vi "Teleop.vi"(10 "Match Info":T2={"Autonomous Elapsed Seconds"=0.0, "TeleOp Elapsed Seconds"=72.02, "Disabled Elapsed Seconds"=100.939, "Visited Autonomous"=FALSE, "Visited TeleOp"=TRUE, "Visited Disabled"=TRUE, "Autonomous Settings"={"Autonomous Style"=enum."Independent", "VI Refnum"=refnum}}, 11 "Call Context":T3=enum."Stop") -> ()   [LabVIEW 2018]
doc: "This VI is called for each enabled TeleOp packet received from the DS. It is typically used to read from joysticks and other inputs and update I/O or setpoints for timed control loops. It should complete and return within 20 milliseconds or risk missing DS packets."
uses:
  <vilib>/Rock Robotics/WPI/DriverStation/WPI_DriverStationDerivedRobotMode.ctl
  <vilib>/Rock Robotics/WPI/DriverStation/WPI_DriverStationMatch Info.ctl
  Elevator/Implementation/Elevator Operations.ctl
  <vilib>/Rock Robotics/WPI/Utilities/WPI_GetSetVariantRefNum.vi
  Elevator/Implementation/Elevator Published Globals.vi
  <vilib>/Rock Robotics/Network Tables/NT Write Boolean.vi
  Framework/Robot Global Data.vi
  Configuration/Constants.vi
  <vilib>/Rock Robotics/Network Tables/NT Write Boolean Array.vi
  <vilib>/Rock Robotics/Network Tables/NT Write Numeric Array.vi
panel:
  in  "Anti-Gravity Elevator":dbl=0.06
  in  "Cluster":T1={"OutakeSpeed"=0.4, "OutakeSpeed Fast"=1.0, "Intake Sens"=1.2, "OutakeSens"=0.7} {"OutakeSpeed Fast" format="%#_13g"; "OutakeSpeed" format="%#_13g"}
  in  "ElevatorheightToSLowMode":dbl=25.0 format="%#_13g"
  in  "ElevatorInterpolate":cluster{"X":dbl, "Y":dbl}[](array[cluster])=[{"X"=0.0, "Y"=0.0}, {"X"=0.05, "Y"=0.0}, {"X"=0.8, "Y"=0.3}, {"X"=1.0, "Y"=1.0}]
  in  "ElevatorheightToSLowerMode":dbl=45.0 format="%#_13g"
  in  "Max dx/dt":dbl=100.0
  in  "Points":cluster{"X":dbl, "Y":dbl}[](array[cluster])=[{"X"=0.0, "Y"=0.0}, {"X"=0.02, "Y"=0.0}, {"X"=0.021, "Y"=0.15}, {"X"=1.0, "Y"=1.0}]
  in  "Drive":enum16{"Cheesy", "Tank"}(ring)
  # "Keep negative"
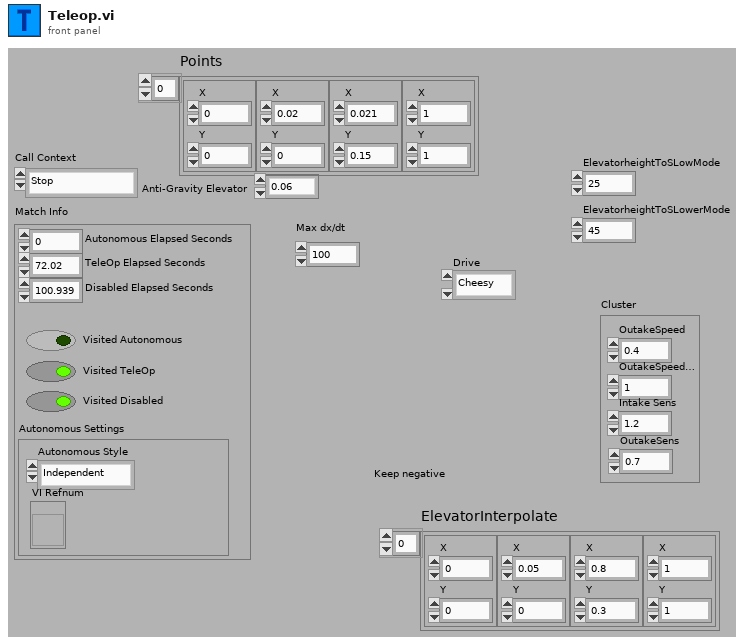
[diagram p1: front panel]
types:
  T1 = cluster{"OutakeSpeed":dbl, "OutakeSpeed Fast":dbl, "Intake Sens":dbl, "OutakeSens":dbl}
  T2 = typedef "WPI_DriverStationMatch Info.ctl" = cluster{"Autonomous Elapsed Seconds":dbl, "TeleOp Elapsed Seconds":dbl, "Disabled Elapsed Seconds":dbl, "Visited Autonomous":bool, "Visited TeleOp":bool, "Visited Disabled":bool, "Autonomous Settings":cluster{"Autonomous Style":enum16{"Iterative", "Independent"}, "VI Refnum":refnum<vi>}}
  T3 = typedef "WPI_DriverStationDerivedRobotMode.ctl" = enum16{"Init", "Execute", "Stop"}
  T4 = typedef "WPI_JoystickDevRef.ctl" = cluster{"Device":T5}
  T5 = typedef "WPI_JoystickDeviceEnum.ctl" = enum16{"USB 0", "USB 1", "USB 2", "USB 3", "USB 4", "USB 5"}
  T6 = typedef "Command Status Info.ctl" = cluster{"Name":string, "Status":T7, "notifier out":T8}
  T7 = typedef "Completion Status.ctl" = enum16{"Successful", "Aborted", "Incomplete"}
  T8 = typedef "Completion Notifier.ctl" = refnum<notifier>
  T9 = typedef "Elevator Operations.ctl" = enum16{"Reserve", "Read Current", "Immediate", "GoToHeight", "StayAtHeight", "LiftForTime"}
  T10 = typedef "Elevator Setpoints.ctl" = cluster{"Operation":T9, "Setpoint":dbl, "Duration":dbl, "Button":bool}
  T11 = cluster{"Current Command":T10, "Command Timing":cluster{"Start Time (ms)":u32, "Iterations":i32}, "Command Arguments":cluster{"Command Info":T6, "Description":string, "Default Command":T10, "queue out":refnum<queue>, "Subsystem Name":string}}
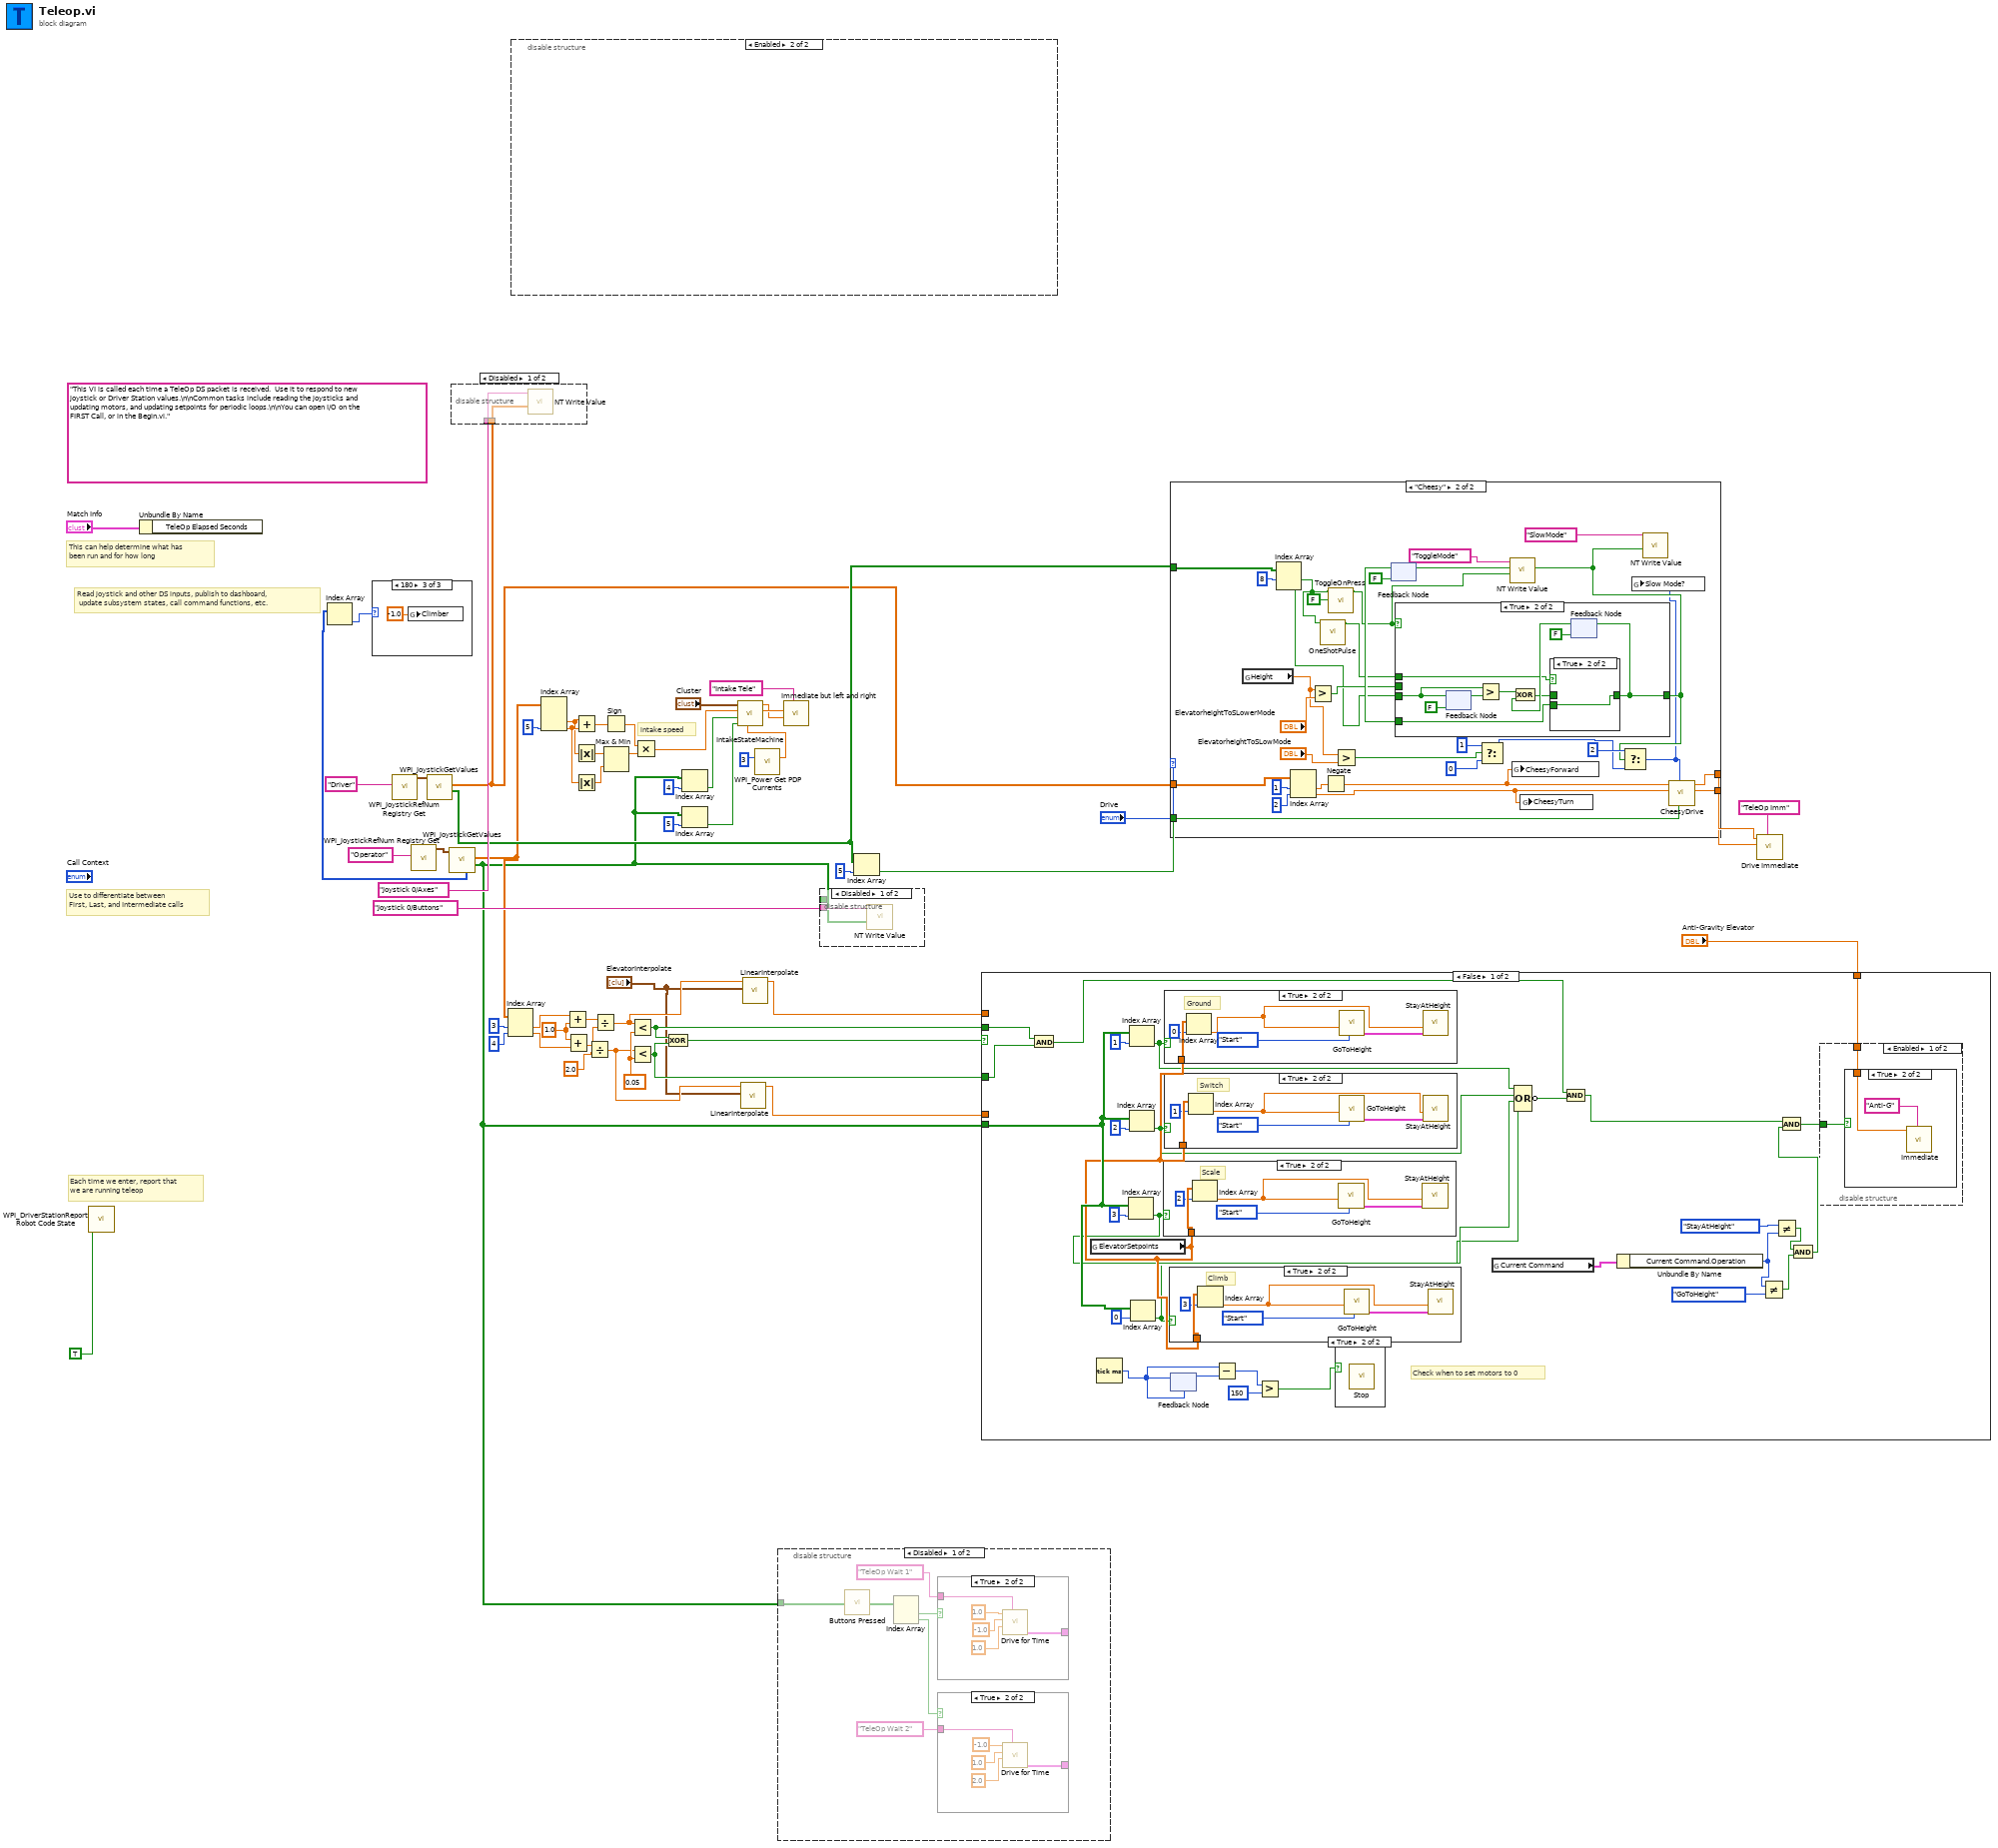
[diagram p0: block diagram]
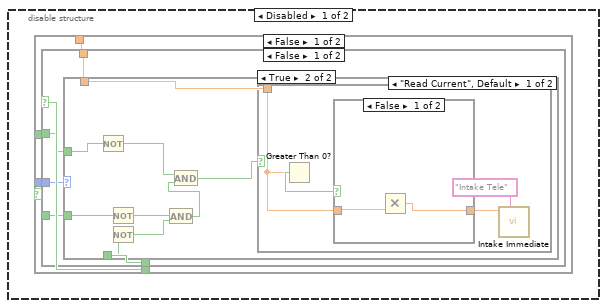
[diagram p2: hidden frame]
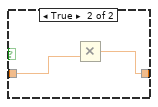
[diagram p4: hidden frame]
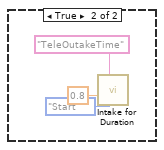
[diagram p6: hidden frame]
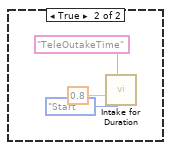
[diagram p7: hidden frame]
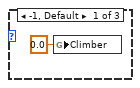
[diagram p8: hidden frame]
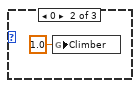
[diagram p9: hidden frame]
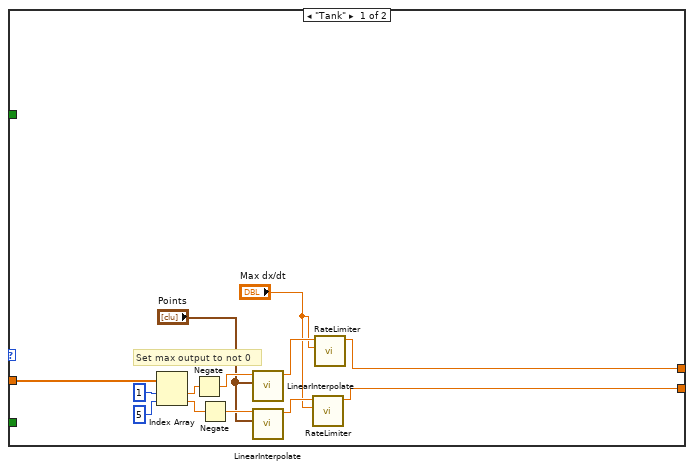
[diagram p12: hidden frame]
diagram:
  w28 = 2.0 ("y")
  w33 = 1.0 ("y")
  w43 = 0.05 ("x")
  (unwired) "This VI is called each time a TeleOp DS packet is received.  Use it to respond to new joystick or Driver Station values.\n\nCommon tasks include reading the joysticks and updating motors, and updating setpoints for periodic loops.\n\nYou can open I/O on the FIRST Call, or in the Begin.vi."
  # "intake speed"
  # "Read joystick and other DS inputs, publish to dashboard,\n update subsystem states, call command functions, etc."
  # "Each time we enter, report that\nwe are running teleop"
  # "Use to differentiate between\nFirst, Last, and Intermediate calls"
  # "This can help determine what has\nbeen run and for how long"
  n1 = call <vilib>:"WPI_DriverStationReport Robot Code State.vi"("TeleOp"=TRUE ("Autonomous")) -> ()  [unwired: 10 in, 1 out]
  n2 = Unbundle By Name("Match Info") -> ()  [unwired: 1 out]
  n3 = call <vilib>:"WPI_JoystickRefNum Registry Get.vi"("refnum name"="Driver") -> ("JoystickDevRef"=w39:T4)  [unwired: 1 in, 9 out]
  n4 = call <vilib>:"WPI_JoystickRefNum Registry Get.vi"("refnum name"="Operator") -> ("JoystickDevRef"=w55:T4)  [unwired: 1 in, 9 out]
  n5 = call <vilib>:"WPI_JoystickGetValues.vi"("JoystickDevRef"=w39) -> ("Buttons"=w37:bool[], "Axes"=w7:dbl[])  [unwired: 6 in, 3 out]
  n6 = call <vilib>:"WPI_JoystickGetValues.vi"("JoystickDevRef"=w55) -> ("Buttons"=w21:bool[], "Axes"=w36:dbl[], "POVs"=w34:i16[])  [unwired: 6 in, 2 out]
  n7 = Index Array(array=w34) -> (element=w12:i16)  [unwired: 1 in]
  n8 = case shown="180" w12 {
    frame -1, Default {
      n9 = global write "Robot Global Data.vi" "Climber"(0.0 ("Climber")) -> ()
    }
    frame 0 {
      n10 = global write "Robot Global Data.vi" "Climber"(1.0 ("Climber")) -> ()
    }
    frame 180 {
      n11 = global write "Robot Global Data.vi" "Climber"(-1.0 ("Climber")) -> ()
    }
  }
  n12 = disable-structure shown="Disabled" {
    disable-tunnel: "Joystick 0/Axes" ("Name") -> [w62 _]
    disable-tunnel: w7 -> [w61 _]
    frame Disabled {
      n13 = call-poly <vilib>:"NT Write Value.vi"("Numeric Array"=w61, "Name"=w62) -> ()  [unwired: 9 in, 1 out]
    }
    frame Enabled {
    }
  }
  n14 = Index Array(array=w36, index #1=3 ("index"), index #2=4 ("index")) -> (element #1=w31:dbl, element #2=w32:dbl)
  n15 = disable-structure shown="Enabled" {
    frame Disabled {
      n16 = case shown="False" {
        selector: _ -> [_ _]
        tunnel: _ -> [w63 _]
        tunnel: _ -> [w66 _]
        tunnel: _ -> [w65 _]
        tunnel: _ -> [w64 _]
        frame False {
          n17 = case shown="False" w63 {
            tunnel: w66 -> [w71 _]
            tunnel: w65 -> [w70 _]
            tunnel: w64 -> [w69 _]
            tunnel: _ -> [w68 _]
            tunnel: w63 -> [w67 _]
            frame False {
              n18 = case shown="\"Read Current\", Default" w69 {
                tunnel: w71 -> [w80 _]
                tunnel: w70 -> [w79 _]
                tunnel: w68 -> [w77 _]
                tunnel: w67 -> [w76 _]
                frame "Read Current", Default {
                  n19 = Not(x=w79) -> (.not. x?=w78:bool)
                  n20 = Not(x=w77) -> (.not. x?=w75:bool)
                  n21 = Not(x=w76) -> (.not. x?=w74:bool)
                  n22 = And(x=w75, y=w74) -> (x .and. y?=w73:bool)
                  n23 = And(x=w78, y=w73) -> (x .and. y?=w72:bool)
                  n24 = case shown="True" w72 {
                    tunnel: w80 -> [_ w81]
                    frame False {
                    }
                    frame True {
                      n25 = Greater Than 0?(x=w81) -> (x > 0?=w83:bool)
                      n26 = case shown="False" w83 {
                        tunnel: w81 -> [w86 w88]
                        tunnel: [w85 w87] -> w82
                        frame False {
                          n27 = Multiply(y=w86) -> (x*y=w85:dbl)  [unwired: 1 in]
                        }
                        frame True {
                          n28 = Multiply(y=w88) -> (x*y=w87:dbl)  [unwired: 1 in]
                        }
                      }
                      n29 = call "Intake Immediate.vi"("Description"="Intake Tele", "Speed"=w82) -> ()  [unwired: 9 in, 1 out]
                    }
                  }
                }
                frame "Intake for Duration" {
                }
              }
            }
            frame True {
              n30 = call "Intake for Duration.vi"("Synchronization"=enum16{"Start", "Wait"}."Start", "Description"="TeleOutakeTime", "Duration (s)"=0.8) -> ()  [unwired: 8 in, 1 out]
            }
          }
        }
        frame True {
          n31 = call "Intake for Duration.vi"("Synchronization"=enum16{"Start", "Wait"}."Start", "Description"="TeleOutakeTime", "Duration (s)"=0.8) -> ()  [unwired: 8 in, 1 out]
        }
      }
    }
    frame Enabled {
    }
  }
  n32 = Index Array(array=w36, index #3=5 ("index")) -> (element #2=w16:dbl, element #3=w17:dbl)  [unwired: 2 in, 1 out]
  n33 = Add(x=w31, y=w33) -> (x+y=w30:dbl)
  n34 = Add(x=w33, y=w32) -> (x+y=w29:dbl)
  n35 = Add(x=w16, y=w17) -> (x+y=w15:dbl)
  n36 = Absolute Value(x=w16) -> (abs(x)=w19:dbl)
  n37 = Absolute Value(x=w17) -> (abs(x)=w18:dbl)
  n38 = Divide(x=w29, y=w28) -> (x/y=w25:dbl)
  n39 = Divide(x=w30, y=w28) -> (x/y=w27:dbl)
  n40 = Sign(1:w15) -> (0:w14:dbl)
  n41 = Max & Min(x=w19, y=w18) -> (max(x,y)=w13:dbl)  [unwired: 1 out]
  n42 = Less?(x=w27, y=w43) -> (x < y?=w42:bool)
  n43 = Less?(x=w25, y=w43) -> (x < y?=w41:bool)
  n44 = Multiply(x=w14, y=w13) -> (x*y=w10:dbl)
  n45 = Exclusive Or(1:w41, 2:w42) -> (0:w52:bool)
  n46 = Index Array(array=w21, index=4) -> (element=w9:bool)
  n47 = Index Array(array=w21, index=5) -> (element=w8:bool)
  n48 = call "LinearInterpolate.vi"("Points"="ElevatorInterpolate", "Value"=w25) -> ("Output"=w24:dbl)  [unwired: 9 in]
  n49 = call "LinearInterpolate.vi"("Points"="ElevatorInterpolate", "Value"=w27) -> ("Output"=w26:dbl)  [unwired: 9 in]
  n50 = call <vilib>:"WPI_Power Get PDP Currents.vi"("PDP Channel"=3) -> ("current (A)"=w1:dbl)  [unwired: 12 in, 2 out]
  n51 = call "IntakeStateMachine.vi"("IntakeCurrent"=w1, "SlowButton"=w8, "FastButton"=w9, "Joystick"=w10, "Cluster"="Cluster") -> ("Left Intake"=w4:dbl, "Right Intake"=w3:dbl)  [unwired: 5 in]
  n52 = disable-structure shown="Disabled" {
    disable-tunnel: w21 -> [w95 _]
    frame Disabled {
      n53 = call "Buttons Pressed.vi"("Button Values"=w95) -> ("Button Presses"=w96:bool[])
      n54 = Index Array(array=w96) -> (element #1=w98:bool, element #2=w97:bool)  [unwired: 2 in]
      n55 = case shown="True" w98 {
        tunnel: [_ w109] -> _
        tunnel: "TeleOp Wait 1" ("Description") -> [_ w108]
        frame False {
        }
        frame True {
          n56 = call "Drive for Time.vi"("Description"=w108, "Seconds"=1.0, "Right Speed"=-1.0, "Left Speed"=1.0) -> ("Command Info Out"=w109:T6)  [unwired: 6 in, 1 out]
        }
      }
      n57 = case shown="True" w97 {
        tunnel: [_ w103] -> _
        tunnel: "TeleOp Wait 2" ("Description") -> [_ w102]
        frame False {
        }
        frame True {
          n58 = call "Drive for Time.vi"("Description"=w102, "Seconds"=2.0, "Right Speed"=1.0, "Left Speed"=-1.0) -> ("Command Info Out"=w103:T6)  [unwired: 6 in, 1 out]
        }
      }
    }
    frame Enabled {
    }
  }
  n59 = call "Immediate but left and right.vi"("Description"="Intake Tele", "Right Speed"=w3, "Left Speed"=w4) -> ()  [unwired: 8 in, 1 out]
  n60 = disable-structure shown="Disabled" {
    disable-tunnel: "Joystick 0/Buttons" ("Name") -> [w112 _]
    disable-tunnel: w21 -> [w111 _]
    frame Disabled {
      n61 = call-poly <vilib>:"NT Write Value.vi"("Boolean Array"=w111, "Name"=w112) -> ()  [unwired: 9 in, 1 out]
    }
    frame Enabled {
    }
  }
  n62 = Index Array(array=w37, index=5) -> (element=w51:bool)
  n63 = case shown="False" w52 {
    tunnel: w21 -> [w130 _]
    tunnel: w42 -> [w136 w168]
    tunnel: w41 -> [w135 w169]
    tunnel: w26 -> [_ w167]
    tunnel: w24 -> [_ w166]
    tunnel: "Anti-Gravity Elevator" -> [w113 _]
    frame False {
      # "Check when to set motors to 0"
      n64 = And(x=w136, y=w135) -> (x .and. y?=w124:bool)
      n65 = global read "Constants.vi" "ElevatorSetpoints"() -> (w129:dbl[])
      n66 = Tick Count (ms)() -> (millisecond timer value=w140:u32)
      n67 = Index Array(array=w130, index=3) -> (element=w126:bool)
      n68 = Index Array(array=w130, index=1) -> (element=w128:bool)
      n69 = Index Array(array=w130, index=2) -> (element=w127:bool)
      n70 = Index Array(array=w130, index=0) -> (element=w125:bool)
      n71 = case shown="True" w126 {
        tunnel: w129 -> [_ w153]
        frame False {
        }
        frame True {
          # "Scale"
          n72 = Index Array(array=w153, index=2) -> (element=w152:dbl)
          n73 = call "GoToHeight.vi"("Synchronization"=enum16{"Start", "Wait"}."Start", "Setpoint"=w152) -> ("Command Info Out"=w154:T6)  [unwired: 9 in]
          n74 = call "StayAtHeight.vi"("Command Info In"=w154, "Setpoint"=w152) -> ()  [unwired: 9 in, 1 out]
        }
      }
      n75 = case shown="True" w128 {
        tunnel: w129 -> [_ w163]
        frame False {
        }
        frame True {
          # "Ground"
          n76 = Index Array(array=w163, index=0) -> (element=w162:dbl)
          n77 = call "GoToHeight.vi"("Synchronization"=enum16{"Start", "Wait"}."Start", "Setpoint"=w162) -> ("Command Info Out"=w164:T6)  [unwired: 9 in]
          n78 = call "StayAtHeight.vi"("Command Info In"=w164, "Setpoint"=w162) -> ()  [unwired: 9 in, 1 out]
        }
      }
      n79 = case shown="True" w127 {
        tunnel: w129 -> [_ w158]
        frame False {
        }
        frame True {
          # "Switch"
          n80 = Index Array(array=w158, index=1) -> (element=w157:dbl)
          n81 = call "GoToHeight.vi"("Synchronization"=enum16{"Start", "Wait"}."Start", "Setpoint"=w157) -> ("Command Info Out"=w159:T6)  [unwired: 9 in]
          n82 = call "StayAtHeight.vi"("Command Info In"=w159, "Setpoint"=w157) -> ()  [unwired: 9 in, 1 out]
        }
      }
      n83 = case shown="True" w125 {
        tunnel: w129 -> [_ w148]
        frame False {
        }
        frame True {
          # "Climb"
          n84 = Index Array(array=w148, index=3) -> (element=w147:dbl)
          n85 = call "GoToHeight.vi"("Synchronization"=enum16{"Start", "Wait"}."Start", "Setpoint"=w147) -> ("Command Info Out"=w149:T6)  [unwired: 9 in]
          n86 = call "StayAtHeight.vi"("Command Info In"=w149, "Setpoint"=w147) -> ()  [unwired: 9 in, 1 out]
        }
      }
      n87 = feedback-in #1(w140) -> ()
      n88 = feedback #1(w140) -> (w141:u32)
      n89 = Subtract(x=w140, y=w141) -> (x-y=w139:u32)
      n90 = Greater?(x=w139, y=u32 150) -> (0:w137:bool)
      n91 = case shown="True" w137 {
        frame False {
        }
        frame True {
          n92 = call "Stop.vi"() -> ()  [unwired: 11 in, 1 out]
        }
      }
      n93 = global read "Elevator Published Globals.vi" "Current Command"() -> (w121:T11)
      n94 = Compound Arithmetic op=OR(w128, w127, w126, w125) -> (invert w114:bool)
      n95 = And(x=w124, y=w114) -> (x .and. y?=w123:bool)
      n96 = Unbundle By Name(w121) -> ("Current Command.Operation"=w119:T9)
      n97 = Not Equal?(x=w119, y=Elevator_Operations."GoToHeight") -> (x != y?=w118:bool)
      n98 = Not Equal?(x=Elevator_Operations."StayAtHeight" ("y"), y=w119) -> (x != y?=w117:bool)
      n99 = And(x=w117, y=w118) -> (x .and. y?=w116:bool)
      n100 = And(x=w123, y=w116) -> (x .and. y?=w115:bool)
      n101 = disable-structure shown="Enabled" {
        disable-tunnel: w115 -> [w143 _]
        disable-tunnel: w113 -> [w142 _]
        frame Enabled {
          n102 = case shown="True" w143 {
            tunnel: w142 -> [_ w145]
            frame False {
            }
            frame True {
              n103 = call "Immediate.vi"("Description"="Anti-G", "Setpoint"=w145) -> ()  [unwired: 9 in, 1 out]
            }
          }
        }
        frame Disabled {
        }
      }
    }
    frame True {
      # "Moves down for up to -.5 speed"
      # "Moves up for up to .5 speed"
      n104 = Not(x=w168) -> (.not. x?=w170:bool)
      n105 = Not(x=w169) -> (.not. x?=w172:bool)
      n106 = And(x=w169, y=w170) -> (x .and. y?=w171:bool)
      n107 = And(x=w172, y=w168) -> (x .and. y?=w173:bool)
      n108 = case shown="True" w173 {
        tunnel: w166 -> [_ w179]
        frame False {
        }
        frame True {
          n109 = Divide(x=w179, y=2.0) -> (x/y=w178:dbl)
          n110 = call "Immediate.vi"("Setpoint"=w178) -> ()  [unwired: 10 in, 1 out]
        }
      }
      n111 = case shown="True" w171 {
        tunnel: w167 -> [_ w176]
        frame False {
        }
        frame True {
          n112 = Divide(x=w176, y=2.0) -> (x/y=w175:dbl)
          n113 = Negate(x=w175) -> (-x=w174:dbl)
          n114 = call "Immediate.vi"("Setpoint"=w174) -> ()  [unwired: 10 in, 1 out]
        }
      }
    }
  }
  n115 = case shown="\"Cheesy\"" "Drive" {
    tunnel: w51 -> [_ w221]
    tunnel: [w184 w222] -> w48
    tunnel: [w182 w223] -> w47
    tunnel: w7 -> [w193 w224]
    tunnel: w37 -> [_ w213]
    frame "Tank" {
      # "Set max output to not 0"
      n116 = Index Array(array=w193, index #1=1 ("index"), index #2=5 ("index")) -> (element #1=w190:dbl, element #2=w189:dbl)
      n117 = Negate(x=w190) -> (-x=w188:dbl)
      n118 = Negate(x=w189) -> (-x=w187:dbl)
      n119 = call "LinearInterpolate.vi"("Points"="Points", "Value"=w188) -> ("Output"=w185:dbl)  [unwired: 9 in]
      n120 = call "LinearInterpolate.vi"("Points"="Points", "Value"=w187) -> ("Output"=w183:dbl)  [unwired: 9 in]
      n121 = call "RateLimiter.vi"("Max dx/dt"="Max dx/dt", "Input"=w183) -> ("Output"=w182:dbl)  [unwired: 9 in]
      n122 = call "RateLimiter.vi"("Max dx/dt"="Max dx/dt", "Input"=w185) -> ("Output"=w184:dbl)  [unwired: 9 in]
    }
    frame "Cheesy" {
      n123 = global read "Elevator Published Globals.vi" "Height"() -> (w202:dbl)
      n124 = Index Array(array=w213, index #1=8 ("index")) -> (element #1=w210:bool, element #2=w208:bool)  [unwired: 1 in]
      n125 = Index Array(array=w224, index #1=1 ("index"), index #2=2 ("index")) -> (element #1=w218:dbl, element #2=w203:dbl)
      n126 = Greater?(x=w202, y="ElevatorheightToSLowerMode") -> (0:w209:bool)
      n127 = call "OneShotPulse.vi"("Input"=w210) -> ("Output"=w212:bool)  [unwired: 10 in]
      n128 = Negate(x=w218) -> (-x=w204:dbl)
      n129 = call "ToggleOnPress.vi"("InitialOuput"=FALSE, "Input"=w210) -> ("Output"=w205:bool)  [unwired: 9 in]
      n130 = Greater?(x=w202, y="ElevatorheightToSLowMode") -> (0:w199:bool)
      n131 = feedback #2(FALSE ("InitialOuput")) -> (w215:bool)
      n132 = case shown="True" w205 {
        tunnel: w209 -> [w225 _]
        tunnel: [w225 w228] -> w195
        tunnel: w208 -> [_ w231]
        tunnel: w215 -> [_ w229]
        tunnel: w212 -> [_ w227]
        frame False {
        }
        frame True {
          n133 = feedback #3(FALSE ("Input")) -> (w235:bool)
          n134 = feedback-in #3(w231) -> ()
          n135 = Greater?(x=w231, y=w235) -> (0:w232:bool)
          n136 = feedback #4(FALSE ("InitialOuput")) -> (w233:bool)
          n137 = Exclusive Or(1:w233, 2:w232) -> (0:w230:bool)
          n138 = case shown="True" w227 {
            tunnel: w230 -> [w236 _]
            tunnel: [w236 w237] -> w228
            tunnel: w229 -> [_ w237]
            frame False {
            }
            frame True {
            }
          }
          n139 = feedback-in #4(w228) -> ()
        }
      }
      n140 = feedback-in #2(w195) -> ()
      n141 = Select(t=1, s=w199, f=0 ("index")) -> (s? t:f=w196:i32)
      n142 = call-poly <vilib>:"NT Write Value.vi"("Boolean"=w205, "Name"="ToggleMode") -> ()  [unwired: 9 in, 1 out]
      n143 = global write "Robot Global Data.vi" "CheesyForward"(w204) -> ()
      n144 = global write "Robot Global Data.vi" "CheesyTurn"(w203) -> ()
      n145 = Select(t=2 ("index"), s=w195, f=w196) -> (s? t:f=w194:i32)
      n146 = global write "Robot Global Data.vi" "Slow Mode?"(w194) -> ()
      n147 = call-poly <vilib>:"NT Write Value.vi"("Boolean"=w195, "Name"="SlowMode") -> ()  [unwired: 9 in, 1 out]
      n148 = call "CheesyDrive.vi"("Quickturn"=w221, "SlowMode"=w194, "Wheel"=w203, "Throttle"=w204) -> ("Right PWM"=w223:dbl, "Left PWM"=w222:dbl)  [unwired: 6 in]
    }
  }
  n149 = call "Drive Immediate.vi"("Description"="TeleOp Imm", "Right Setpoint"=w47, "Left Setpoint"=w48) -> ()  [unwired: 8 in, 1 out]
